vi "onInterruptEndLoop.vi"(8 "error in (no error)":errorcluster, 10 "model in":refnum<class "IModel.lvclass">, 11 "FaultState in":refnum<class "FaultState.lvclass">) -> (0 "error out":errorcluster, 2 "model out":refnum<class "IModel.lvclass">, 3 "FaultState out":refnum<class "FaultState.lvclass">)   [LabVIEW 2012, in "States.lvlib" / "FaultState.lvclass"]
uses:
  FaultState.lvclass
  IModel/IModel.lvclass
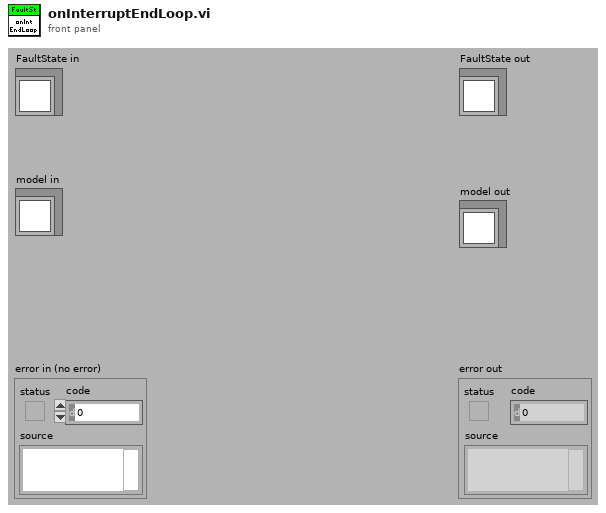
[diagram p1: front panel]
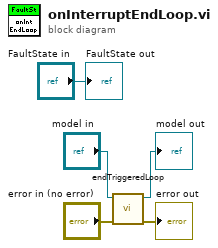
[diagram p0: block diagram]
diagram:
  n1 = call-dynamic "endTriggeredLoop.vi"("error in (no error)"="error in (no error)", "IModel in"="model in") -> ("error out"=→"error out":errorcluster, "IModel out"=→"model out":refnum<class "IModel.lvclass">)  [unwired: 8 in]
  "FaultState out" <- "FaultState in"
